vi "ini_read_variant.vi"(7 "section":string, 8 "error in":errorcluster, 9 "default":variant, 10 "key":string, 11 "refnum in":T1) -> (0 "error out":errorcluster, 1 "variant out":variant, 2 "found?":bool, 3 "refnum out":T1)   [LabVIEW 2018]
uses:
  <vilib>/Utility/config.llb/Config Data RefNum.ctl
  <vilib>/Utility/config.llb/Read Key (String).vi
  <vilib>/Utility/config.llb/NI_LVConfig.lvlib
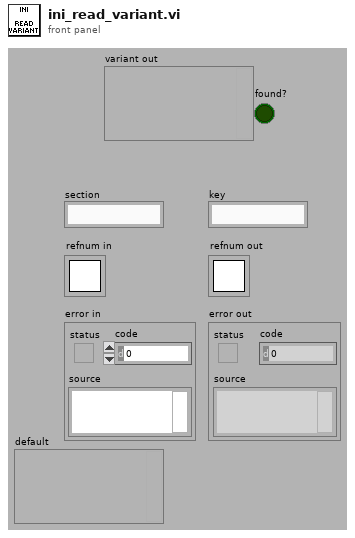
[diagram p1: front panel]
types:
  T1 = typedef "NI_LVConfig.lvlib/Config Data RefNum.ctl" = refnum<k1>
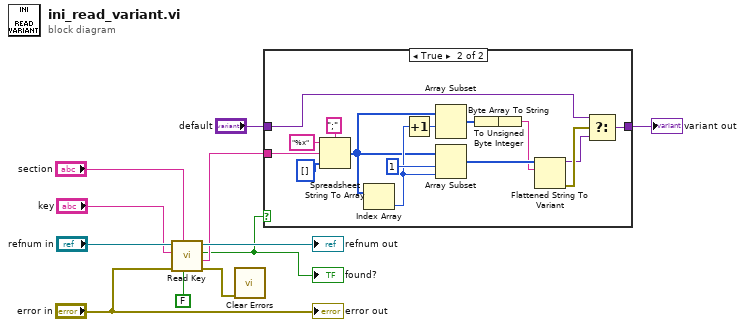
[diagram p0: block diagram]
diagram:
  n1 = call-poly <vilib>:"Read Key.vi"("read raw string? (F)"=FALSE, "section"="section", "error in (no error)"="error in", "key"="key", "refnum"="refnum in") -> ("error out"=w6:errorcluster, "value"=w5:string, "found?"=w4:bool, "refnum out"=→"refnum out":T1)  [unwired: 3 in]
  "found?" <- w4
  n2 = call <vilib>:"Clear Errors.vi"("error in (no error)"=w6) -> ()  [unwired: 5 in, 2 out]
  n3 = case shown="True" w4 {
    tunnel: w5 -> [_ w28]
    tunnel: [w12 w16] -> w2
    tunnel: "default" -> [w12 w14]
    frame False {
    }
    frame True {
      n4 = Spreadsheet String To Array(delimiter (Tab)=";", format string="%x", spreadsheet string=w28, array type (2D Dbl)=u16[] []) -> (array=w21:u16[])
      n5 = Index Array(array=w21) -> (element=w22:u16)  [unwired: 1 in]
      n6 = Increment(x=w22) -> (x+1=w23:u16)
      n7 = Array Subset(array=w21, index=w23) -> (w20:u16[])  [unwired: 1 in]
      n8 = Array Subset(array=w21, index=1, length=w22) -> (w18:u16[])
      n9 = To Unsigned Byte Integer(number=w20) -> (unsigned 8bit integer=w19:u8[])
      n10 = Byte Array To String(unsigned byte array=w19) -> (string=w17:string)
      n11 = Flattened String To Variant(6:w17, 7:w18) -> (0:w15:errorcluster, 3:w13:variant)  [unwired: 1 in]
      n12 = Select(t=w14, s=w15, f=w13) -> (s? t:f=w16:variant)
    }
  }
  "variant out" <- w2
  "error out" <- "error in"
